vi "PWM sweep host.vi"() -> ()   [LabVIEW 2013]
uses:
  <vilib>/userdefined/High Color/nirio_resource_hc.ctl
  <vilib>/Utility/error.llb/DialogType.ctl
  <vilib>/DAQmx/read.llb/DAQmx Read (Analog 1D Wfm NChan NSamp).vi
  <vilib>/rvi/interface/common/niFpgaWaitOnOcc.vi
  <vilib>/DAQmx/write.llb/DAQmx Write (Analog 1D DBL 1Chan NSamp).vi
  <vilib>/DAQmx/create/channels.llb/DAQmx Create Channel (AI-Voltage-Basic).vi
  <vilib>/DAQmx/configure/timing.llb/DAQmx Timing (Sample Clock).vi
  <vilib>/DAQmx/configure/task.llb/DAQmx Configure Logging (TDMS).vi
  <vilib>/DAQmx/create/channels.llb/DAQmx Create Channel (AO-Voltage-Basic).vi
  <vilib>/DAQmx/configure/trigger.llb/DAQmx Start Trigger (Digital Edge).vi
  <vilib>/DAQmx/configure/trigger.llb/DAQmx Start Trigger (Analog Edge).vi
  <vilib>/DAQmx/configure/trigger.llb/DAQmx Reference Trigger (Digital Edge).vi
  <vilib>/DAQmx/configure/trigger.llb/DAQmx Reference Trigger (Analog Edge).vi
  <vilib>/FPGAPlugInAG/PCIe-1473R-LX110/niLvFpga_Open_PCIe-1473R-LX110.vi
  <vilib>/rvi/interface/common/dynamic/niFpgaDynamicAddResources.vi
  <vilib>/DAQmx/miscellaneous.llb/DAQmx Fill In Error Info.vi
  <vilib>/Utility/error.llb/Error Cluster From Error Code.vi
  <vilib>/rvi/errors/niLvFpgaAdjustHostInterfaceError.vi
  <vilib>/FPGAPlugInAG/Dynamic/niLvFpga_Close_Dynamic.vi
  <vilib>/rvi/interface/nirviOpenFPGA/nirviOpenFPGA.xnode
  FPGA Bitfiles/PWMTest_FPGATarget2_4TTL.lvbitx
  FPGA VIs/PWM FPGA test2.vi
  <vilib>/rvi/interface/nirviReadWriteControl/nirviReadWriteControl.xnode
  <vilib>/rvi/interface/nirviCloseFPGA/nirviCloseFPGA.xnode
  <resource>/objmgr/daqmx.rc
  NiFpgaLv.dll
  <vilib>/rvi/interface/Simulation/niFpgaSimulationCallBeginRW.vi
panel:
  in  "TTL 4":bool=TRUE
  in  "TTL 3":bool=TRUE
  in  "numRandomLoops":i32=2000 caption="(-1 = inf)"
  out "Current\nDuty Cycle":dbl=0.9944999999999999
  out "sweep stop":bool=TRUE
  out "loop duration (ms)":dbl=5.0
  out "sweep loops":u32=255
  out "loop #":u32=255
  in  "Duty Cycle Step":dbl=0.0039
  in  "Duty Cycle Mode":T1(ring)=enum."Sweep Duty Cycle"
  in  "Auto AO?":bool=TRUE
  in  "Manual AO (V)":dbl=1.0
  in  "Max Voltage Out":dbl=5.0
  in  "Min Voltage Out":dbl
  in  "Physical Channel(s)":tag="Dev1/ao0"
  in  "Trigger Type":T2(tab)
  in  "Edge":i32(ring)=10280 items=["Rising"=10280, "Falling"=10171]
  in  "Digital Trigger Source":tag
  in  "Level (V)":dbl format="%0.2f"
  in  "Hysteresis (V)":dbl
  in  "Slope":i32(ring)=10280 items=["Rising"=10280, "Falling"=10171]
  in  "Analog Trigger Source":string="APFI0"
  in  "Digital Ref Trigger Source":tag
  in  "Edge 2":i32(ring)=10280 items=["Rising"=10280, "Falling"=10171]
  in  "Pre-Trigger Samples":u32
  in  "Analog Ref Trigger Source":string="APFI0"
  in  "Slope 2":i32(ring)=10280 items=["Rising"=10280, "Falling"=10171]
  in  "Level (V) 2":dbl format="%0.2f"
  in  "Pre-Trigger Samples 2":u32
  out "Waveform Graph":waveform(dbl)[](graph)=[{"t0"=timestamp(3472482620.069274 s since 1904-01-01), "dt"=2.4999999999999957e-05, "Y"=[4.952422825991433, 4.953410049292613, 4.952093751557871, 4.952422825991433, 4.952093751557871, 4.952751900425078, 4.952422825991433, 4.953080974858804, 4.952093751557871, 4.952751900425078, 4.952093751557871, 4.952751900425078, 4.952751900425078, 4.952751900425078, 4.952093751557871, 4.952422825991433, 4.952422825991433, 4.953080974858804, 4.952751900425078, 4.952422825991433, 4.952093751557871, 4.952093751557871, 4.952751900425078, 4.952422825991433, 4.953080974858804, 4.952422825991433, 4.953410049292613, 4.952422825991433, 4.952751900425078, 4.951764677124391, 4.952751900425078, 4.952422825991433, 4.953080974858804, 4.952422825991433, 4.952751900425078, 4.952422825991433, 4.952751900425078, 4.952751900425078, 4.952751900425078, 4.952751900425078, 4.952422825991433, 4.952422825991433, 4.953080974858804, 4.953080974858804, 4.952751900425078, 4.952422825991433, 4.952422825991433, 4.952751900425078, 4.952422825991433, 4.952751900425078, 4.952422825991433, 4.953080974858804, 4.952422825991433, 4.952422825991433, 4.951764677124391, 4.952751900425078, 4.952422825991433, 4.953080974858804, 4.952751900425078, 4.952422825991433, 4.952751900425078, 4.952751900425078, 4.953410049292613, 4.953080974858804, 4.951764677124391, 4.952093751557871, 4.952751900425078, 4.952422825991433, 4.952751900425078, 4.952422825991433, 4.952751900425078, 4.952093751557871, 4.952751900425078, 4.952093751557871, 4.953410049292613, 4.952751900425078, 4.953080974858804, 4.951764677124391, 4.953080974858804, 4.952093751557871, 4.952422825991433, 4.952093751557871, 4.952751900425078, 4.952093751557871, 4.952751900425078, 4.952422825991433, 4.952422825991433, 4.952751900425078, 4.972825441033057, 4.971838217717298, 4.972496366594388, 4.971838217717298, 4.972167292155802, 4.972167292155802, 4.972167292155802, 4.971838217717298, 4.972167292155802, 4.972496366594388, 4.972167292155802, 4.972825441033057, 4.971838217717298, 4.972825441033057, 4.972167292155802, 4.972167292155802, 4.971180068840539, 4.972825441033057, 4.972167292155802, 4.972496366594388, 4.971838217717298, 4.971838217717298, 4.971838217717298, 4.972496366594388, 4.972167292155802, 4.972496366594388, 4.971838217717298, 4.972167292155802, 4.971838217717298, 4.972496366594388, 4.972167292155802, 4.972167292155802, 4.971838217717298, 4.971838217717298, 4.971509143278878, 4.972167292155802, 4.972167292155802, 4.972496366594388, 4.972167292155802, 4.971838217717298, 4.971838217717298, 4.971180068840539, 4.972825441033057, 4.971838217717298, 4.972496366594388, 4.972167292155802, 4.972496366594388, 4.971838217717298, 4.972496366594388, 4.972167292155802, 4.971838217717298, 4.971838217717298, 4.972167292155802, 4.971838217717298, 4.972167292155802, 4.971838217717298, 4.972496366594388, 4.971838217717298, 4.972167292155802, 4.971838217717298, 4.972167292155802, 4.971838217717298, 4.972167292155802, 4.972496366594388, 4.971838217717298, 4.972167292155802, 4.971509143278878, 4.972167292155802, 4.971838217717298, 4.972496366594388, 4.971509143278878, 4.971838217717298, 4.972167292155802, 4.972496366594388, 4.972496366594388, 4.972496366594388, 4.972167292155802, 4.972496366594388, 4.971838217717298, 4.972496366594388, 4.971838217717298, 4.972496366594388, 4.971838217717298, 4.971509143278878, 4.972496366594388, 4.971838217717298, 4.972167292155802, 4.972167292155802, 4.972496366594388, 4.971509143278878, 4.971838217717298, 4.971509143278878, 4.972496366594388, 4.971509143278878, 4.972167292155802, 4.971509143278878, 4.972167292155802, 4.971838217717298, 4.972496366594388, 4.972167292155802, 4.972167292155802, 4.971838217717298, 4.972167292155802, 4.971838217717298, 4.972167292155802, 4.971838217717298, 4.972496366594388, 4.971509143278878, 4.971838217717298, 4.971838217717298, 4.972167292155802, 4.972167292155802], "attributes"=variant("NI_ChannelName"=variant(string "Dev1/ai1"), "NI_UnitDescription"=variant(string "Volts"))}, {"t0"=timestamp(3472482620.069279 s since 1904-01-01), "dt"=2.4999999999999957e-05, "Y"=[4.952093751557871, 4.951764677124391, 4.951764677124391, 4.952093751557871, 4.952093751557871, 4.952093751557871, 4.951764677124391, 4.952751900425078, 4.952093751557871, 4.951764677124391, 4.951106528257678, 4.951764677124391, 4.951435602690993, 4.951435602690993, 4.951435602690993, 4.951106528257678, 4.950777453824444, 4.950777453824444, 4.950777453824444, 4.950777453824444, 4.951106528257678, 4.951106528257678, 4.951106528257678, 4.950448379391293, 4.950777453824444, 4.950777453824444, 4.951106528257678, 4.950448379391293, 4.951106528257678, 4.950448379391293, 4.950777453824444, 4.950777453824444, 4.951106528257678, 4.950777453824444, 4.950777453824444, 4.951106528257678, 4.950777453824444, 4.950448379391293, 4.951106528257678, 4.950777453824444, 4.950448379391293, 4.950777453824444, 4.950777453824444, 4.950448379391293, 4.950777453824444, 4.950777453824444, 4.950777453824444, 4.950777453824444, 4.950448379391293, 4.950448379391293, 4.951106528257678, 4.951435602690993, 4.951764677124391, 4.952093751557871, 4.951764677124391, 4.952093751557871, 4.951764677124391, 4.952422825991433, 4.952422825991433, 4.952093751557871, 4.952093751557871, 4.952422825991433, 4.952093751557871, 4.952093751557871, 4.952093751557871, 4.952422825991433, 4.952093751557871, 4.951764677124391, 4.952093751557871, 4.952093751557871, 4.952093751557871, 4.952422825991433, 4.952093751557871, 4.951764677124391, 4.952422825991433, 4.952093751557871, 4.952093751557871, 4.952422825991433, 4.952093751557871, 4.952093751557871, 4.951764677124391, 4.951764677124391, 4.951764677124391, 4.951435602690993, 4.951435602690993, 4.951106528257678, 4.951435602690993, 4.951106528257678, 4.951106528257678, 4.951106528257678, 4.950777453824444, 4.951106528257678, 4.951106528257678, 4.950777453824444, 4.950777453824444, 4.950448379391293, 4.951106528257678, 4.950777453824444, 4.951106528257678, 4.951106528257678, 4.951106528257678, 4.951106528257678, 4.951106528257678, 4.951106528257678, 4.950777453824444, 4.951106528257678, 4.950777453824444, 4.951435602690993, 4.950777453824444, 4.951106528257678, 4.950448379391293, 4.950777453824444, 4.950448379391293, 4.950777453824444, 4.950448379391293, 4.950448379391293, 4.950448379391293, 4.950448379391293, 4.950448379391293, 4.951106528257678, 4.955713570331579, 4.959333389115242, 4.962295059036557, 4.96492765452777, 4.966573026712457, 4.967560250024257, 4.968876547774478, 4.968876547774478, 4.969534696650083, 4.96920562221224, 4.970192845526018, 4.970192845526018, 4.970850994402283, 4.970521919964109, 4.970850994402283, 4.970192845526018, 4.970192845526018, 4.970192845526018, 4.971180068840539, 4.970192845526018, 4.971509143278878, 4.970850994402283, 4.970850994402283, 4.970850994402283, 4.970850994402283, 4.970521919964109, 4.971180068840539, 4.970850994402283, 4.970850994402283, 4.970850994402283, 4.970850994402283, 4.970850994402283, 4.970850994402283, 4.971180068840539, 4.971180068840539, 4.971180068840539, 4.970521919964109, 4.971180068840539, 4.971180068840539, 4.970850994402283, 4.970521919964109, 4.970850994402283, 4.970850994402283, 4.970850994402283, 4.970850994402283, 4.970521919964109, 4.970521919964109, 4.970850994402283, 4.970521919964109, 4.970850994402283, 4.971180068840539, 4.971180068840539, 4.971180068840539, 4.971180068840539, 4.970850994402283, 4.971180068840539, 4.970850994402283, 4.971180068840539, 4.971509143278878, 4.970850994402283, 4.970521919964109, 4.970192845526018, 4.970850994402283, 4.970850994402283, 4.970521919964109, 4.970850994402283, 4.970850994402283, 4.970850994402283, 4.971180068840539, 4.970521919964109, 4.971180068840539, 4.970521919964109, 4.971180068840539, 4.971180068840539, 4.971180068840539, 4.971180068840539, 4.971180068840539, 4.970850994402283, 4.971180068840539, 4.971180068840539], "attributes"=variant("NI_ChannelName"=variant(string "Dev1/ai5"), "NI_UnitDescription"=variant(string "Volts"))}, {"t0"=timestamp(3472482620.069284 s since 1904-01-01), "dt"=2.4999999999999957e-05, "Y"=[4.952422825991433, 4.951764677124391, 4.952093751557871, 4.952093751557871, 4.952093751557871, 4.952422825991433, 4.951764677124391, 4.952422825991433, 4.952093751557871, 4.952093751557871, 4.951764677124391, 4.951764677124391, 4.951435602690993, 4.951764677124391, 4.951106528257678, 4.951106528257678, 4.950777453824444, 4.951106528257678, 4.950448379391293, 4.951106528257678, 4.951106528257678, 4.951435602690993, 4.950777453824444, 4.950777453824444, 4.951106528257678, 4.950777453824444, 4.950777453824444, 4.951106528257678, 4.951106528257678, 4.950777453824444, 4.950448379391293, 4.951106528257678, 4.951106528257678, 4.950777453824444, 4.951106528257678, 4.951106528257678, 4.951435602690993, 4.950777453824444, 4.951106528257678, 4.950777453824444, 4.951106528257678, 4.951106528257678, 4.951435602690993, 4.951435602690993, 4.951764677124391, 4.952093751557871, 4.951764677124391, 4.952093751557871, 4.952093751557871, 4.952093751557871, 4.952093751557871, 4.952422825991433, 4.952422825991433, 4.952751900425078, 4.952093751557871, 4.952093751557871, 4.952093751557871, 4.952093751557871, 4.952422825991433, 4.952093751557871, 4.952751900425078, 4.952093751557871, 4.952422825991433, 4.952422825991433, 4.952093751557871, 4.952422825991433, 4.952422825991433, 4.952422825991433, 4.951764677124391, 4.952422825991433, 4.952093751557871, 4.952422825991433, 4.952422825991433, 4.952422825991433, 4.952422825991433, 4.952422825991433, 4.952422825991433, 4.952093751557871, 4.952093751557871, 4.952093751557871, 4.952093751557871, 4.952093751557871, 4.951435602690993, 4.951764677124391, 4.951764677124391, 4.951435602690993, 4.951435602690993, 4.951435602690993, 4.951435602690993, 4.951106528257678, 4.951106528257678, 4.951435602690993, 4.951435602690993, 4.951106528257678, 4.951106528257678, 4.950777453824444, 4.951106528257678, 4.951106528257678, 4.951106528257678, 4.951106528257678, 4.951435602690993, 4.951106528257678, 4.951106528257678, 4.950777453824444, 4.950777453824444, 4.951106528257678, 4.951435602690993, 4.951106528257678, 4.951106528257678, 4.950777453824444, 4.951106528257678, 4.950777453824444, 4.950119304958224, 4.950777453824444, 4.950448379391293, 4.950448379391293, 4.950448379391293, 4.951106528257678, 4.950777453824444, 4.950448379391293, 4.954068198160478, 4.958346165809619, 4.961965984600526, 4.964269505654473, 4.965914877838335, 4.967231175586908, 4.968218398899203, 4.96920562221224, 4.969534696650083, 4.970521919964109, 4.970192845526018, 4.970521919964109, 4.970521919964109, 4.970521919964109, 4.971180068840539, 4.970850994402283, 4.971180068840539, 4.970850994402283, 4.971180068840539, 4.970850994402283, 4.971180068840539, 4.971180068840539, 4.970850994402283, 4.970850994402283, 4.971180068840539, 4.970521919964109, 4.971509143278878, 4.971180068840539, 4.971509143278878, 4.971180068840539, 4.971180068840539, 4.970850994402283, 4.971180068840539, 4.971180068840539, 4.971838217717298, 4.971509143278878, 4.971509143278878, 4.971180068840539, 4.970850994402283, 4.970521919964109, 4.971509143278878, 4.971509143278878, 4.971838217717298, 4.971509143278878, 4.970850994402283, 4.971180068840539, 4.970850994402283, 4.971180068840539, 4.971509143278878, 4.971838217717298, 4.971180068840539, 4.971180068840539, 4.971180068840539, 4.971838217717298, 4.971180068840539, 4.971509143278878, 4.971180068840539, 4.971509143278878, 4.971838217717298, 4.971180068840539, 4.971180068840539, 4.970521919964109, 4.970850994402283, 4.970850994402283, 4.971180068840539, 4.971180068840539, 4.971180068840539, 4.971509143278878, 4.971180068840539, 4.970850994402283, 4.971509143278878, 4.971180068840539, 4.971509143278878, 4.971509143278878, 4.970850994402283, 4.971180068840539, 4.971509143278878, 4.971180068840539, 4.971509143278878, 4.970850994402283], "attributes"=variant("NI_ChannelName"=variant(string "Dev1/ai6"), "NI_UnitDescription"=variant(string "Volts"))}, {"t0"=timestamp(3472482620.069289 s since 1904-01-01), "dt"=2.4999999999999957e-05, "Y"=[4.128091617075155, 4.128091617075155, 4.127762542834709, 4.1284206913156725, 4.1284206913156725, 4.1284206913156725, 4.1290788397969225, 4.1284206913156725, 4.1290788397969225, 4.1290788397969225, 4.1290788397969225, 4.129407914037656, 4.129736988278461, 4.130066062519338, 4.130066062519338, 4.130066062519338, 4.130066062519338, 4.130395136760287, 4.130066062519338, 4.130724211001308, 4.130724211001308, 4.130724211001308, 4.130724211001308, 4.131053285242401, 4.130724211001308, 4.131053285242401, 4.130724211001308, 4.131053285242401, 4.131053285242401, 4.131382359483567, 4.131382359483567, 4.131711433724804, 4.131382359483567, 4.132040507966113, 4.131711433724804, 4.1323695822074935, 4.132698656448946, 4.132698656448946, 4.1323695822074935, 4.1323695822074935, 4.1323695822074935, 4.1323695822074935, 4.1323695822074935, 4.132698656448946, 4.133027730690472, 4.133027730690472, 4.132698656448946, 4.133356804932069, 4.133685879173738, 4.133027730690472, 4.134344027657292, 4.134344027657292, 4.134344027657292, 4.134673101899177, 4.134344027657292, 4.134344027657292, 4.134673101899177, 4.135002176141135, 4.135002176141135, 4.135002176141135, 4.135002176141135, 4.135989398867439, 4.135660324625266, 4.135989398867439, 4.135660324625266, 4.135660324625266, 4.135989398867439, 4.136318473109684, 4.136318473109684, 4.136318473109684, 4.136318473109684, 4.136318473109684, 4.136318473109684, 4.136976621594392, 4.1373056958368535, 4.136976621594392, 4.136976621594392, 4.137634770079387, 4.137634770079387, 4.137634770079387, 4.137634770079387, 4.137963844321993, 4.137634770079387, 4.137963844321993, 4.13829291856467, 4.137963844321993, 4.13829291856467, 4.138621992807421, 4.13829291856467, 4.138621992807421, 4.138951067050242, 4.13829291856467, 4.138621992807421, 4.138621992807421, 4.138951067050242, 4.138621992807421, 4.138951067050242, 4.138951067050242, 4.139609215536103, 4.138951067050242, 4.139609215536103, 4.139609215536103, 4.139280141293137, 4.139609215536103, 4.139609215536103, 4.139280141293137, 4.139280141293137, 4.139609215536103, 4.139609215536103, 4.139938289779141, 4.139609215536103, 4.139938289779141, 4.139938289779141, 4.140267364022252, 4.140267364022252, 4.140596438265434, 4.140267364022252, 4.140925512508689, 4.140596438265434, 4.140925512508689, 4.143887180701227, 4.145532551921828, 4.146848848899608, 4.146848848899608, 4.147506997388931, 4.1478360716337015, 4.148165145878544, 4.148823294368444, 4.148823294368444, 4.148823294368444, 4.149481442858634, 4.1498105171038375, 4.150139591349113, 4.1504686655944605, 4.1498105171038375, 4.150139591349113, 4.15079773983988, 4.151126814085372, 4.151455888330937, 4.152114036822282, 4.151455888330937, 4.151784962576573, 4.151784962576573, 4.152114036822282, 4.152443111068063, 4.152772185313917, 4.152772185313917, 4.152772185313917, 4.153101259559842, 4.15343033380584, 4.153101259559842, 4.1537594080519105, 4.1537594080519105, 4.154088482298053, 4.154417556544268, 4.154417556544268, 4.154088482298053, 4.154417556544268, 4.154746630790555, 4.154417556544268, 4.155404779283345, 4.155075705036914, 4.155404779283345, 4.155733853529849, 4.155404779283345, 4.155404779283345, 4.156062927776426, 4.155733853529849, 4.1563920020230745, 4.156721076269795, 4.156721076269795, 4.157050150516588, 4.156721076269795, 4.157050150516588, 4.157050150516588, 4.157708299010391, 4.157708299010391, 4.157708299010391, 4.157708299010391, 4.157379224763454, 4.158037373257401, 4.157708299010391, 4.158037373257401, 4.158037373257401, 4.158366447504484, 4.158695521751639, 4.158695521751639, 4.158695521751639, 4.159024595998866, 4.1593536702461655, 4.159024595998866, 4.159024595998866, 4.1593536702461655, 4.1593536702461655, 4.159682744493537, 4.160011818740981, 4.160011818740981, 4.160340892988498, 4.160340892988498, 4.160669967236086], "attributes"=variant("NI_ChannelName"=variant(string "Dev1/ai7"), "NI_UnitDescription"=variant(string "Volts"))}, {"t0"=timestamp(3472482620.069294 s since 1904-01-01), "dt"=2.4999999999999957e-05, "Y"=[9.901384858496838, 9.900726706228475, 9.903359315305384, 9.900068553960688, 9.902372086900463, 9.899081325560086, 9.901713934631236, 9.902043010765778, 9.905004695983129, 9.903359315305384, 9.901055782362585, 9.89875224942684, 9.900068553960688, 9.902372086900463, 9.901384858496838, 9.902043010765778, 9.903688391440644, 9.903030239170265, 9.89875224942684, 9.903359315305384, 9.900068553960688, 9.905662848255234, 9.899410401693476, 9.901713934631236, 9.897435944895296, 9.901384858496838, 9.899410401693476, 9.90039763009451, 9.89809409716078, 9.90039763009451, 9.898423173293738, 9.900726706228475, 9.900068553960688, 9.900068553960688, 9.901384858496838, 9.900726706228475, 9.90039763009451, 9.89875224942684, 9.89973947782701, 9.900726706228475, 9.902372086900463, 9.899081325560086, 9.897765021027967, 9.89480333583911, 9.899410401693476, 9.897765021027967, 9.902043010765778, 9.90039763009451, 9.899081325560086, 9.896448716498147, 9.90039763009451, 9.901713934631236, 9.903688391440644, 9.901384858496838, 9.903030239170265, 9.897435944895296, 9.89973947782701, 9.900068553960688, 9.903359315305384, 9.901055782362585, 9.903030239170265, 9.90039763009451, 9.900726706228475, 9.901384858496838, 9.903359315305384, 9.902043010765778, 9.902043010765778, 9.902372086900463, 9.896119640366052, 9.900726706228475, 9.901713934631236, 9.904346543711599, 9.902701163035292, 9.902372086900463, 9.900068553960688, 9.901384858496838, 9.900726706228475, 9.905991924391504, 9.900068553960688, 9.902043010765778, 9.903359315305384, 9.900726706228475, 9.903030239170265, 9.901384858496838, 9.903030239170265, 9.903030239170265, 9.901713934631236, 9.902701163035292, 9.905333772119109, 9.902701163035292, 9.902701163035292, 9.902043010765778, 9.89973947782701, 9.899410401693476, 9.901384858496838, 9.90039763009451, 9.901713934631236, 9.899410401693476, 9.903359315305384, 9.89710686876277, 9.901055782362585, 9.896448716498147, 9.903030239170265, 9.899081325560086, 9.900726706228475, 9.896448716498147, 9.899410401693476, 9.899410401693476, 9.901713934631236, 9.90039763009451, 9.899081325560086, 9.898423173293738, 9.89809409716078, 9.899081325560086, 9.89809409716078, 9.903359315305384, 9.900068553960688, 9.89875224942684, 9.895790564234101, 9.901713934631236, 9.902372086900463, 9.917180513110358, 9.92047127452996, 9.92705279741242, 9.928369101995836, 9.93462154879859, 9.93396339650111, 9.938899538746288, 9.935608777245893, 9.937912310294653, 9.935279701096649, 9.939228614897122, 9.938241386445053, 9.9405449195019, 9.940215843350488, 9.94186122410899, 9.939228614897122, 9.940215843350488, 9.940215843350488, 9.941203071805157, 9.943835681023957, 9.940215843350488, 9.941532147957002, 9.9405449195019, 9.940215843350488, 9.939886767199223, 9.94317752871839, 9.937912310294653, 9.940215843350488, 9.937912310294653, 9.939886767199223, 9.9385704625956, 9.941203071805157, 9.939228614897122, 9.939886767199223, 9.939228614897122, 9.941532147957002, 9.938899538746288, 9.940215843350488, 9.9405449195019, 9.941203071805157, 9.937912310294653, 9.938241386445053, 9.940873995653456, 9.937254157994285, 9.94317752871839, 9.9385704625956, 9.939886767199223, 9.937254157994285, 9.941532147957002, 9.938899538746288, 9.94317752871839, 9.9395576910481, 9.941203071805157, 9.938241386445053, 9.940215843350488, 9.937912310294653, 9.943506604871102, 9.939228614897122, 9.941203071805157, 9.9385704625956, 9.941203071805157, 9.939886767199223, 9.94186122410899, 9.941203071805157, 9.941203071805157, 9.938899538746288, 9.939228614897122, 9.940873995653456, 9.940873995653456, 9.9425193764134, 9.940215843350488, 9.9405449195019, 9.9385704625956, 9.941532147957002, 9.9395576910481, 9.9425193764134, 9.940215843350488, 9.941203071805157, 9.936925081844318], "attributes"=variant("NI_ChannelName"=variant(string "Dev1/ai16"), "NI_UnitDescription"=variant(string "Volts"))}]
  in  "TDMS File Path":path=path "F:/Live_Data/20140113 FPGA WBA DAC Test/20140113 FPGA WBA DAC Test Duty Cycle Sweeps/20140113 FPGA WBA DAC Test 5msLoop 0039step 255loops 40KHz Trial10.tdms"
  in  "Logging Mode":i32(ring)=15842 items=["Off"=10231, "Log and Read"=15842]
  in  "numSamples/loop":i32=200
  in  "Sample Rate":dbl=40000.0
  in  "Sample Clock Source":tag="OnboardClock"
  out "Actual Sample Rate":dbl=40000.0 format="%0.2f"
  in  "Terminal Configuration":i32(ring)=10083 items=["default"=-1, "RSE"=10083, "NRSE"=10078, "Differential"=10106, "Pseudodifferential"=12529]
  in  "Max Voltage":dbl=10.0
  in  "Min Voltage":dbl=-10.0
  in  "Physical Channel":tag="Dev1/ai1, Dev1/ai5:7, Dev1/ai16"
  in  "TTL 2":bool=TRUE
  in  "TTL 1":bool=TRUE
  in  "ISO Out 2":bool
  in  "ISO Out 1":bool
  in  "ISO Out 0":bool
  in  "resource name":T3="rio0" caption="RIO Device"
  out "error out":errorcluster
  out "Running?":bool
  in  "Stop":bool
  in  "Carrier Frequency (Hz)":dbl(slide)=4000.0 scale=0.0..10000.0 scale format="%#_6p"
  in  "Duty cycle":dbl(slide)=0.4050464807436919 scale=0.0..1.0
  # "Analog Output"
  # "Output"
  # "Analog Inputs"
  # "Acquired Data"
  # "Channel Settings"
  # "Trigger Settings"
  # "To configure and use a start trigger you must have the necessary tab selected above.  Not all hardware supports triggering--refer to your device documentation for more info."
  # "Logging Settings"
  # "Timing Settings"
  # "Channel Settings"
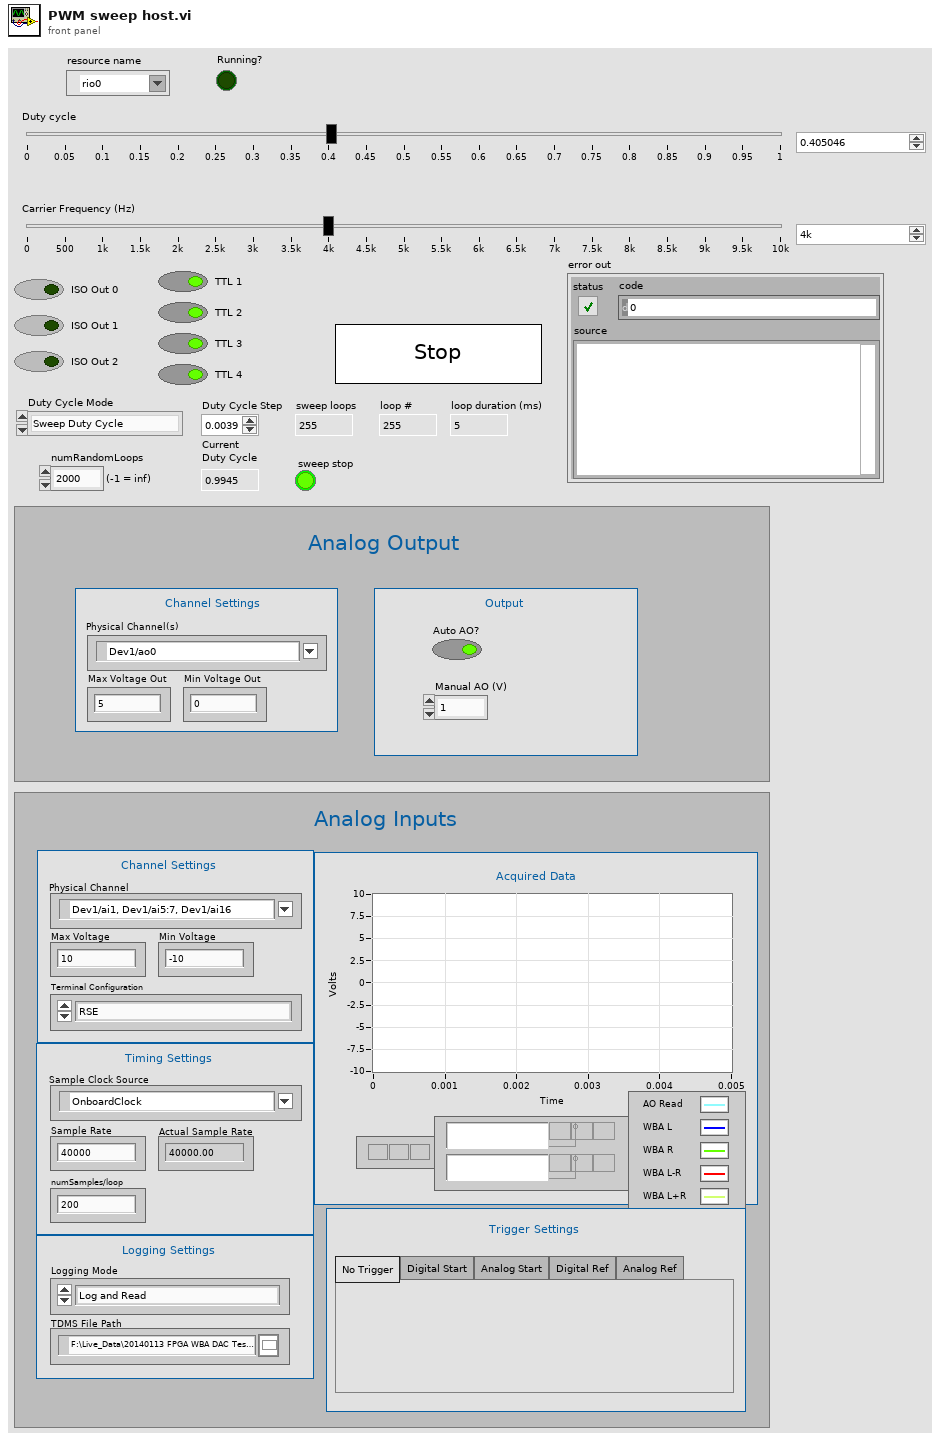
[diagram p1: front panel]
types:
  T1 = enum8{"Manual Duty Cycle", "Sweep Duty Cycle", "Random Duty Cycle"}
  T2 = enum32{"No Trigger", "Digital Start", "Analog Start", "Digital Ref", "Analog Ref"}
  T3 = typedef "nirio_resource_hc.ctl" = tag
  T4 = typedef "DialogType.ctl" = u16
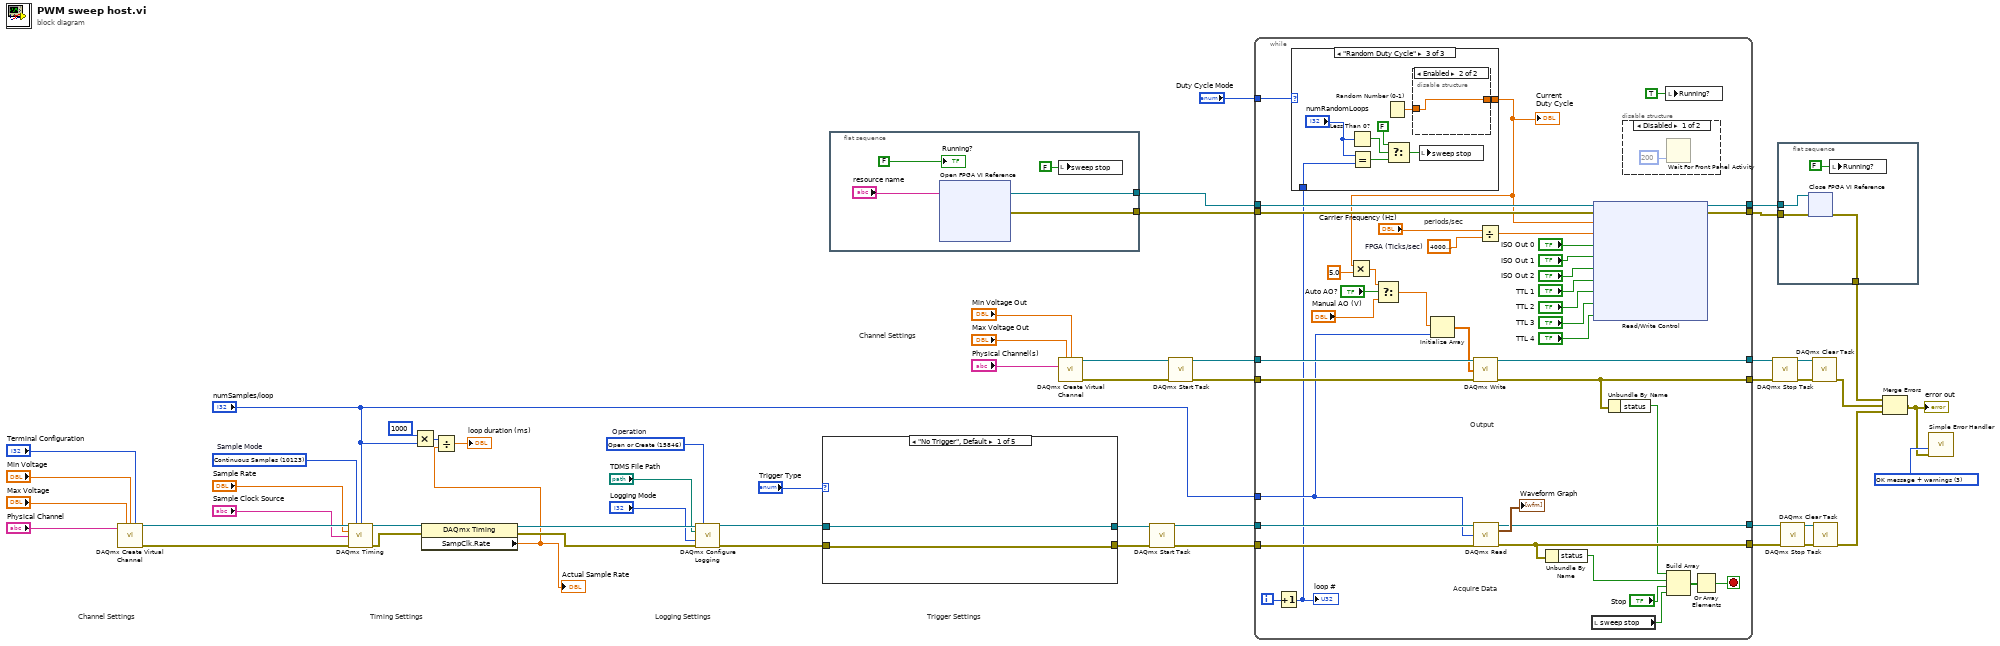
[diagram p0: block diagram]
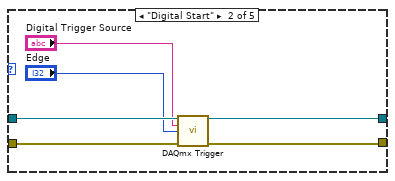
[diagram p2: hidden frame]
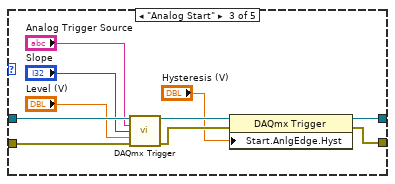
[diagram p3: hidden frame]
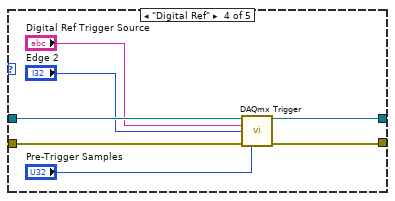
[diagram p4: hidden frame]
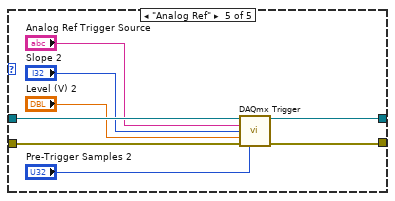
[diagram p5: hidden frame]
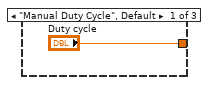
[diagram p6: hidden frame]
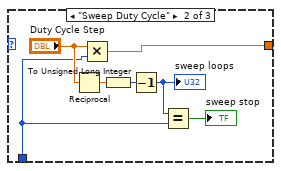
[diagram p7: hidden frame]
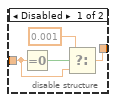
[diagram p8: hidden frame]
diagram:
  w29 = T4 3 items=["no dialog", "OK message", "continue or stop message", "OK message + warnings", "continue/stop + warnings"] ("type of dialog (OK msg:1)")
  w42 = 15846 items=["Open"=10437, "Open or Create"=15846, "Create or Replace"=15847, "Create"=15848]  # Operation
  w47 = 10123 items=["Finite Samples"=10178, "Continuous Samples"=10123, "Hardware Timed Single Point"=12522]  # Sample Mode
  # "Channel Settings"
  # "Trigger Settings"
  # "Timing Settings"
  # "Channel Settings"
  # "Logging Settings"
  n1 = call-poly <vilib>:"DAQmx Create Virtual Channel.vi"("maximum value"="Max Voltage", "minimum value"="Min Voltage", "input terminal configuration"="Terminal Configuration", "physical channels"="Physical Channel") -> ("task out"=w45:refnum<k21>, "error out"=w46:errorcluster)  [unwired: 10 in]
  n2 = call-poly <vilib>:"DAQmx Timing.vi"("task/channels in"=w45, "sample mode"=w47, "samples per channel"="numSamples/loop", "rate"="Sample Rate", "source"="Sample Clock Source", "error in"=w46) -> ("task out"=w49:refnum<k21>, "error out"=w48:errorcluster)  [unwired: 8 in]
  n3 = Multiply(x=1000, y="numSamples/loop") -> (x*y=w8:i32)
  n4 = property class="DAQmx Timing"(reference=w49, error in=w48) -> (reference out=w44:refnum<k21>, error out=w43:errorcluster, "SampClk.Rate"=w3:dbl)
  "Actual Sample Rate" <- w3
  n5 = Divide(x=w8, y=w3) -> (x/y=→"loop duration (ms)":dbl)
  n6 = call-poly <vilib>:"DAQmx Configure Logging.vi"("task/channels in"=w44, "operation"=w42, "file path"="TDMS File Path", "logging mode"="Logging Mode", "error in"=w43) -> ("task out"=w41:refnum<k21>, "error out"=w40:errorcluster)  [unwired: 9 in]
  n7 = case shown="\"No Trigger\", Default" "Trigger Type" {
    tunnel: w41 -> [w55 w61 w71 w78 w86]
    tunnel: w40 -> [w54 w60 w70 w77 w85]
    tunnel: [w55 w59 w68 w76 w80] -> w39
    tunnel: [w54 w58 w67 w75 w81] -> w38
    frame "No Trigger", Default {
    }
    frame "Digital Start" {
      n8 = call-poly <vilib>:"DAQmx Trigger.vi"("task/channels in"=w61, "source"="Digital Trigger Source", "edge"="Edge", "error in"=w60) -> ("task out"=w59:refnum<k21>, "error out"=w58:errorcluster)  [unwired: 10 in]
    }
    frame "Analog Start" {
      n9 = call-poly <vilib>:"DAQmx Trigger.vi"("task/channels in"=w71, "source"="Analog Trigger Source", "slope"="Slope", "level"="Level (V)", "error in"=w70) -> ("task out"=w66:refnum<k21>, "error out"=w65:errorcluster)  [unwired: 9 in]
      n10 = property class="DAQmx Trigger"(reference=w66, error in=w65, "Start.AnlgEdge.Hyst"="Hysteresis (V)") -> (reference out=w68:refnum<k21>, error out=w67:errorcluster)
    }
    frame "Digital Ref" {
      n11 = call-poly <vilib>:"DAQmx Trigger.vi"("task/channels in"=w78, "source"="Digital Ref Trigger Source", "edge"="Edge 2", "error in"=w77, "pretrigger samples per channel"="Pre-Trigger Samples") -> ("task out"=w76:refnum<k21>, "error out"=w75:errorcluster)  [unwired: 9 in]
    }
    frame "Analog Ref" {
      n12 = call-poly <vilib>:"DAQmx Trigger.vi"("task/channels in"=w86, "source"="Analog Ref Trigger Source", "slope"="Slope 2", "level"="Level (V) 2", "error in"=w85, "pretrigger samples per channel"="Pre-Trigger Samples 2") -> ("task out"=w80:refnum<k21>, "error out"=w81:errorcluster)  [unwired: 8 in]
    }
  }
  n13 = flat-sequence {
    tunnel: [w91] -> w53
    tunnel: [w90] -> w52
    frame #0 {
      n14 = xnode "Open FPGA VI Reference"("resource name"="resource name") -> ("FPGA VI Reference Out"=w91:refnum<k20>, "error out"=w90:errorcluster)  [unwired: 1 in]
      n15 = local write "sweep stop"(FALSE ("sweep stop")) -> ()
      "Running?" <- FALSE ("Running?")
    }
  }
  n16 = call-poly <vilib>:"DAQmx Create Virtual Channel.vi"("maximum value"="Max Voltage Out", "minimum value"="Min Voltage Out", "physical channels"="Physical Channel(s)") -> ("task out"=w19:refnum<k21>, "error out"=w18:errorcluster)  [unwired: 11 in]
  n17 = call <vilib>:"DAQmx Start Task.vi"("task/channels in"=w39, "error in"=w38) -> ("task out"=w28:refnum<k21>, "error out"=w27:errorcluster)  [unwired: 12 in]
  n18 = call <vilib>:"DAQmx Start Task.vi"("task/channels in"=w19, "error in"=w18) -> ("task out"=w15:refnum<k21>, "error out"=w14:errorcluster)  [unwired: 12 in]
  n19 = while {
    tunnel: w53 -> [w132]
    tunnel: w52 -> [w131]
    tunnel: [w127] -> w51
    tunnel: [w126] -> w50
    tunnel: "numSamples/loop" -> [w106]
    tunnel: w28 -> [w118]
    tunnel: w27 -> [w117]
    tunnel: [w116] -> w26
    tunnel: [w115] -> w25
    tunnel: w15 -> [w114]
    tunnel: w14 -> [w113]
    tunnel: [w112] -> w13
    tunnel: [w111] -> w12
    tunnel: "Duty Cycle Mode" -> [w99]
    i -> [w97]
    stop <- w119 stop-if-true
    w129 = 40000000.0  # FPGA (Ticks/sec)
    # "Output"
    # "Acquire Data"
    # "periods/sec"
    n20 = Increment(x=w97) -> (x+1=w96:i32)
    "loop #" <- w96
    n21 = case shown="\"Random Duty Cycle\"" w99 {
      tunnel: ["Duty cycle" w140 w142] -> w98
      tunnel: w96 -> [_ w137 w144]
      frame "Manual Duty Cycle", Default {
      }
      frame "Sweep Duty Cycle" {
        n22 = Reciprocal(x="Duty Cycle Step") -> (1/x=w138:dbl)
        n23 = Multiply(x="Duty Cycle Step", y=w137) -> (x*y=w140:dbl)
        n24 = To Unsigned Long Integer(number=w138) -> (unsigned 32bit integer=w136:u32)
        n25 = Decrement(x=w136) -> (x-1=w135:u32)
        "sweep loops" <- w135
        n26 = Equal?(x=w135, y=w137) -> (x = y?=→"sweep stop":bool)
      }
      frame "Random Duty Cycle" {
        n27 = Less Than 0?(x="numRandomLoops") -> (x < 0?=w148:bool)
        n28 = Equal?(x="numRandomLoops", y=w144) -> (x = y?=w143:bool)
        n29 = Random Number (0-1)() -> (number: 0 to 1=w141:dbl)
        n30 = Select(t=FALSE ("sweep stop"), s=w148, f=w143) -> (s? t:f=w147:bool)
        n31 = disable-structure shown="Enabled" {
          disable-tunnel: [w152 w153] -> w142
          disable-tunnel: w141 -> [w151 w153]
          frame Disabled {
            n32 = Equal To 0?(x=w151) -> (x = 0?=w150:bool)
            n33 = Select(t=0.001, s=w150, f=w151) -> (s? t:f=w152:dbl)
          }
          frame Enabled {
          }
        }
        n34 = local write "sweep stop"(w147) -> ()
      }
    }
    "Current\nDuty Cycle" <- w98
    n35 = Multiply(x=w98, y=5.0) -> (x*y=w101:dbl)
    n36 = Select(t=w101, s="Auto AO?", f="Manual AO (V)") -> (s? t:f=w103:dbl)
    n37 = Initialize Array(w103, w106) -> (w105:dbl[])
    n38 = call-poly <vilib>:"DAQmx Write.vi"("task/channels in"=w114, "data"=w105, "error in"=w113) -> ("task out"=w112:refnum<k21>, "error out"=w111:errorcluster)  [unwired: 10 in, 1 out]
    n39 = call-poly <vilib>:"DAQmx Read.vi"("task/channels in"=w118, "number of samples per channel"=w106, "error in"=w117) -> ("task out"=w116:refnum<k21>, "data"=→"Waveform Graph":waveform(dbl)[], "error out"=w115:errorcluster)  [unwired: 10 in]
    n40 = Divide(x="Carrier Frequency (Hz)", y=w129) -> (x/y=w128:dbl)
    n41 = Unbundle By Name(w115) -> ("status"=w109:bool)
    n42 = local read "sweep stop"() -> (w95:bool)
    n43 = xnode "Read/Write Control"("FPGA VI Reference In"=w132, "error in"=w131, "duty cycle (periods)"=w98, "frequency (periods/tick)"=w128, "ISO Out 0"="ISO Out 0", "ISO Out 1"="ISO Out 1", "ISO Out 2"="ISO Out 2", "TTL 1"="TTL 1", "TTL 2"="TTL 2", "TTL 3"="TTL 3", "TTL 4"="TTL 4") -> ("FPGA VI Reference Out"=w126:refnum<k20>, "error out"=w127:errorcluster)
    n44 = Unbundle By Name(w111) -> ("status"=w108:bool)
    n45 = disable-structure shown="Disabled" {
      frame Disabled {
        n46 = Wait For Front Panel Activity(1:200 ("timeout ms (-1 never timeout)")) -> ()  [unwired: 2 in, 1 out]
      }
      frame Enabled {
      }
    }
    n47 = local write "Running?"(TRUE ("Running?")) -> ()
    n48 = Build Array(w108, w109, "Stop", w95) -> (w107:bool[])
    n49 = Or Array Elements(Boolean array=w107) -> (logical OR=w119:bool)
  }
  n50 = call <vilib>:"DAQmx Stop Task.vi"("task/channels in"=w13, "error in"=w12) -> ("task out"=w17:refnum<k21>, "error out"=w16:errorcluster)  [unwired: 12 in]
  n51 = flat-sequence {
    tunnel: w51 -> [w158]
    tunnel: w50 -> [w157]
    tunnel: [w155] -> w11
    frame #0 {
      n52 = xnode "Close FPGA VI Reference"("FPGA VI Reference In"=w157, "error in"=w158) -> ("error out"=w155:errorcluster)
      n53 = local write "Running?"(FALSE ("Running?")) -> ()
    }
  }
  n54 = call <vilib>:"DAQmx Stop Task.vi"("task/channels in"=w26, "error in"=w25) -> ("task out"=w30:refnum<k21>, "error out"=w31:errorcluster)  [unwired: 12 in]
  n55 = call <vilib>:"DAQmx Clear Task.vi"("task in"=w17, "error in"=w16) -> ("error out"=w10:errorcluster)  [unwired: 13 in]
  n56 = call <vilib>:"DAQmx Clear Task.vi"("task in"=w30, "error in"=w31) -> ("error out"=w24:errorcluster)  [unwired: 13 in]
  n57 = Merge Errors(w11, w10, w24) -> (w23:errorcluster)
  "error out" <- w23
  n58 = call <vilib>:"Simple Error Handler.vi"("type of dialog (OK msg:1)"=w29, "error in (no error)"=w23) -> ()  [unwired: 3 in, 5 out]
